vi "gxml_TimeCheck.vi"(7 "error in":errorcluster, 9 "Time String":string, 10 "Item Name":string) -> (0 "error out":errorcluster)   [LabVIEW 2011, in "Third Party VIs.lvlib" / "GXML.lvlib"]
uses:
  <vilib>/regexp/Match Regular Expression.xnode
  GXML.lvlib
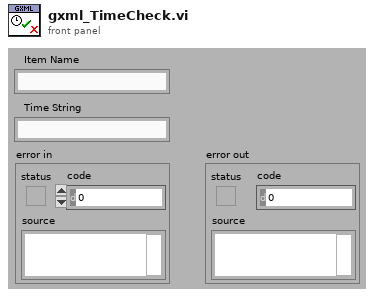
[diagram p1: front panel]
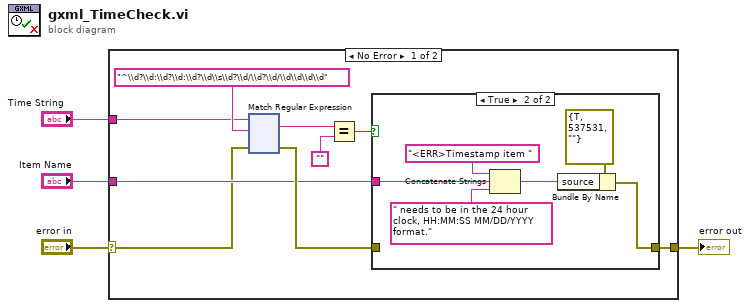
[diagram p0: block diagram]
diagram:
  n1 = case shown="No Error" "error in" {
    selector: "error in" -> [w5 w132]
    tunnel: "Time String" -> [w12 _]
    tunnel: "Item Name" -> [w7 _]
    tunnel: [w6 w132] -> w2
    frame No Error {
      n2 = xnode "Match Regular Expression"("input string"=w12, "regular expression"="^\\d?\\d:\\d?\\d:\\d?\\d\\s\\d?\\d/\\d?\\d/\\d\\d\\d\\d", "error in"=w5) -> ("whole match"=w11:string, "error out"=w8:errorcluster)  [unwired: 3 in, 3 out]
      n3 = Equal?(x=w11, y="") -> (x = y?=w9:bool)
      n4 = case shown="True" w9 {
        tunnel: [w14 w15] -> w6
        tunnel: w8 -> [w14 _]
        tunnel: w7 -> [_ w19]
        frame False {
        }
        frame True {
          n5 = Concatenate Strings("<ERR>Timestamp item " ("string"), w19, " needs to be in the 24 hour clock, HH:MM:SS MM/DD/YYYY format." ("string")) -> (w16:string)
          n6 = Bundle By Name(cluster=errorcluster {"status"=TRUE, "code"=537531, "source"=""} ("error out"), "source"=w16) -> (w15:errorcluster)
        }
      }
    }
    frame Error {
    }
  }
  "error out" <- w2
